vi "Exercises FM Modulation.vi"(8 "错误输入（无错误）":errorcluster, 9 "采样间隔(s)":dbl, 10 "FM 频偏(Hz)":dbl, 11 "数据输入":waveform(dbl)) -> (0 "错误输出":errorcluster, 2 "FM 调制信号(频域)":cluster{"f0":dbl, "df":dbl, "magnitude":dbl[]}(graph)={"f0"=-99999.99999999999, "df"=1.5258789062499998, "magnitude"=[]}, 3 "FM 调制信号(时域)":waveform(cdb) caption="输出波形")   [LabVIEW 2015]
uses:
  <vilib>/measure/NI_MAPro.lvlib
  <vilib>/measure/maresamp.llb/Resample Waveform (single shot).vi
  <vilib>/measure/maspectr.llb/FFT Power Spectrum and PSD for 1 Chan (CDB).vi
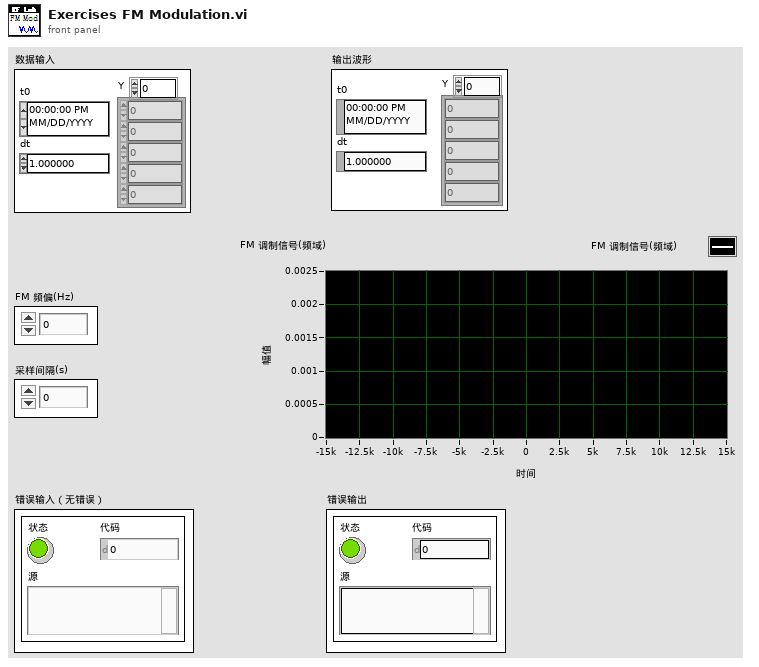
[diagram p1: front panel]
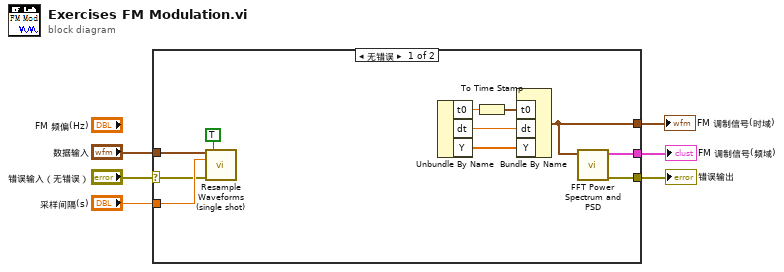
[diagram p0: block diagram]
diagram:
  n1 = case shown="无错误" "错误输入（无错误）" {
    selector: "错误输入（无错误）" -> [w7 w18]
    tunnel: "数据输入" -> [w17 _]
    tunnel: "采样间隔(s)" -> [w16 _]
    tunnel: [w15 _] -> w4
    tunnel: [w14 w18] -> w3
    tunnel: [w13 _] -> w2
    frame No Error {
      n2 = call-poly <vilib>:"Resample Waveforms (single shot).vi"("waveform in"=w17, "open interval? (F)"=TRUE, "dt"=w16, "error in (no error)"=w7) -> ()  [unwired: 8 in, 4 out]
      n3 = Unbundle By Name() -> ("t0"=w11:dbl, "dt"=w10:dbl, "Y"=w9:cdb[])  [unwired: 1 in]
      n4 = To Time Stamp(1:w11) -> (0:w12:timestamp)
      n5 = Bundle By Name("t0"=w12, "dt"=w10, "Y"=w9) -> (w13:waveform(cdb))  [unwired: 1 in]
      n6 = call-poly <vilib>:"FFT Power Spectrum and PSD.vi"("time signal"=w13) -> ("error out"=w14:errorcluster, "Power Spectrum / PSD"=w15:cluster{"f0":dbl, "df":dbl, "magnitude":dbl[]})  [unwired: 7 in, 2 out]
    }
    frame Error {
    }
  }
  "错误输出" <- w3
  "FM 调制信号(频域)" <- w4
  "FM 调制信号(时域)" <- w2
